vi "ATF_PID_V1.0.vi"() -> ()   [LabVIEW 2022 SP3]
panel:
  in  "Monitor":u16=1
  out "Boolean 783":bool
  out "C_FM_39":dbl format="%.2g"
  out "F_EPV_41":bool
  out "C_FM_9":dbl format="%.2g"
  in  "EXIT":bool
  out "F_PT_SC":dbl format="%.2g"
  out "Boolean 7":bool
  out "F_RTD_SC":dbl format="%.2g"
  out "F_PT_42":dbl format="%.2g"
  out "Boolean 781":bool
  out "Boolean 412":bool
  out "Boolean 201":bool
  out "F_PT_47":dbl format="%.2g"
  out "F_RTD_47":dbl format="%.2g"
  out "Boolean 959":bool
  out "Boolean 952":bool
  out "Boolean 780":bool
  out "Boolean 951":bool
  out "Boolean 950":bool
  out "Boolean 941":bool
  out "Boolean 945":bool
  out "Boolean 942":bool
  out "C_LS_LOX_Tank 23":u16(slide) scale=0.0..100.0
  out "G_PT_68":dbl format="%.2g"
  out "C_LS_LOX_Tank 24":u16(slide) scale=0.0..100.0
  out "M_PT_89":dbl format="%.2g"
  out "Boolean 779":bool
  out "Boolean 778":bool
  out "C_EPV_6":bool
  out "C_EPV_6 HSS":bool
  out "C_RTD_5":dbl format="%.2g"
  out "C_PT_5":dbl format="%.2g"
  out "Boolean 777":bool
  out "Boolean 776":bool
  out "C_EPV_13":bool
  out "C_EPV_13 HSS":bool
  out "Boolean 775":bool
  out "Boolean 845":bool
  out "Boolean 844":bool
  out "Boolean 774":bool
  out "Boolean 773":bool
  out "Boolean 873":bool
  out "Boolean 772":bool
  out "Boolean 771":bool
  out "Boolean 770":bool
  out "Boolean 769":bool
  out "Boolean 767":bool
  out "Boolean 766":bool
  out "F_EPV_45":bool
  out "F_EPV_45 HSS":bool
  out "Boolean 765":bool
  out "Boolean 727":bool
  out "Boolean 724":bool
  out "G_PT_72":dbl format="%.2g"
  out "M_PT_93":dbl format="%.2g"
  out "Boolean 1002":bool
  out "Boolean 998":bool
  out "Boolean 872":bool
  out "Boolean 871":bool
  out "Boolean 870":bool
  out "Boolean 862":bool
  out "Boolean 861":bool
  out "Boolean 860":bool
  out "Boolean 859":bool
  out "Boolean 830":bool
  out "I_PT_1":dbl format="%.2g"
  out "I_PT_2":dbl format="%.2g"
  out "E_PT_P2":dbl format="%.2g"
  out "E_PT_P1":dbl format="%.2g"
  out "Boolean 764":bool
  out "Boolean 763":bool
  out "N_EPV_8":bool
  out "Boolean 762":bool
  out "Boolean 761":bool
  out "Boolean 856":bool
  out "Boolean 843":bool
  out "C_PT_189":dbl format="%.2g"
  out "Boolean 791":bool
  out "Boolean 385":bool
  out "Boolean 212":bool
  out "Boolean 760":bool
  out "Boolean 759":bool
  out "Boolean 758":bool
  out "Boolean 757":bool
  out "Boolean 754":bool
  out "Boolean 1076":bool
  out "Boolean 1075":bool
  out "Boolean 958":bool
  out "Boolean 1074":bool
  out "Boolean 1072":bool
  out "Boolean 1073":bool
  out "Boolean 726":bool
  out "Boolean 901":bool
  out "Boolean 1071":bool
  out "Boolean 1033":bool
  out "Boolean 1027":bool
  out "Boolean 411":bool
  out "Boolean 897":bool
  out "Boolean 1070":bool
  out "Boolean 1069":bool
  out "Boolean 1042":bool
  out "Boolean 410":bool
  out "Boolean 1068":bool
  out "Boolean 1067":bool
  out "Boolean 1066":bool
  out "Boolean 1041":bool
  out "Boolean 1016":bool
  out "Boolean 896":bool
  out "Boolean 409":bool
  out "Boolean 1039":bool
  out "Boolean 1015":bool
  out "Boolean 1011":bool
  out "Boolean 1009":bool
  out "Boolean 982":bool
  out "Boolean 1065":bool
  out "Boolean 400":bool
  out "Boolean 408":bool
  out "N_PT_131":dbl format="%.2g"
  out "N_PT_193":dbl format="%.2g"
  out "N_PT_142":dbl format="%.2g"
  out "Boolean 894":bool
  out "Boolean 1063":bool
  out "Boolean 394":bool
  out "Boolean 393":bool
  out "Boolean 1058":bool
  out "Boolean 1018":bool
  out "Boolean 983":bool
  out "Boolean 1064":bool
  out "Boolean 981":bool
  out "Boolean 980":bool
  out "Boolean 979":bool
  out "Boolean 978":bool
  out "Boolean 1062":bool
  out "Boolean 1061":bool
  out "Boolean 977":bool
  out "Boolean 976":bool
  out "Boolean 975":bool
  out "Boolean 1060":bool
  out "Boolean 1059":bool
  out "Boolean 383":bool
  out "Boolean 1057":bool
  out "Boolean 391":bool
  out "Boolean 974":bool
  out "Boolean 883":bool
  out "Boolean 841":bool
  out "Boolean 864":bool
  out "Boolean 854":bool
  out "Boolean 846":bool
  out "Boolean 788":bool
  out "Boolean 796":bool
  out "Boolean 795":bool
  out "Boolean 789":bool
  out "Boolean 1056":bool
  out "Boolean 1055":bool
  out "Boolean 1054":bool
  out "Boolean 1053":bool
  out "Boolean 1052":bool
  out "Boolean 1051":bool
  out "Boolean 1050":bool
  out "Boolean 1049":bool
  out "Boolean 1048":bool
  out "Boolean 1047":bool
  out "Boolean 1046":bool
  out "Boolean 1045":bool
  out "Boolean 1044":bool
  out "Boolean 407":bool
  out "Boolean 1043":bool
  out "Boolean 957":bool
  out "Boolean 956":bool
  out "Boolean 955":bool
  out "Boolean 954":bool
  out "Boolean 953":bool
  out "Boolean 893":bool
  out "Boolean 969":bool
  out "Boolean 968":bool
  out "Boolean 967":bool
  out "Boolean 406":bool
  out "Boolean 966":bool
  out "Boolean 964":bool
  out "N_PT_118":dbl format="%.2g"
  out "Boolean 869":bool
  out "Boolean 1038":bool
  out "Boolean 972":bool
  out "Boolean 971":bool
  out "Boolean 970":bool
  out "Boolean 965":bool
  out "Boolean 868":bool
  out "Boolean 1037":bool
  out "Boolean 1036":bool
  out "Boolean 1035":bool
  out "Boolean 1034":bool
  out "N_PT_102":dbl format="%.2g"
  out "N_PT_107":dbl format="%.2g"
  out "Boolean 1032":bool
  out "Boolean 986":bool
  out "Boolean 1026":bool
  out "Boolean 1025":bool
  out "N_PT_149":dbl format="%.2g"
  out "Boolean 899":bool
  out "Boolean 985":bool
  out "Boolean 1024":bool
  out "Boolean 1023":bool
  out "Boolean 919":bool
  out "Boolean 918":bool
  out "Boolean 855":bool
  out "Boolean 800":bool
  out "Boolean 1022":bool
  out "Boolean 1021":bool
  out "Boolean 1020":bool
  out "Boolean 1019":bool
  out "Boolean 934":bool
  out "Boolean 835":bool
  out "Boolean 815":bool
  out "N_PT_201":dbl format="%.2g"
  out "Boolean 1007":bool
  out "Boolean 993":bool
  out "Boolean 984":bool
  out "Boolean 992":bool
  out "Boolean 991":bool
  out "M_PT_83":dbl format="%.2g"
  out "G_PT_63":dbl format="%.2g"
  out "N_PT_178":dbl format="%.2g"
  out "Boolean 847":bool
  out "Boolean 836":bool
  out "Boolean 211":bool
  out "Boolean 739":bool
  out "Boolean 802":bool
  out "M_EPV_90 HSS":bool
  out "G_EPV_69":bool
  out "M_EPV_90":bool
  out "G_EPV_69 HSS":bool
  out "Boolean 1017":bool
  out "Boolean 1013":bool
  out "Boolean 1010":bool
  out "Boolean 888":bool
  out "Boolean 398":bool
  out "Boolean 405":bool
  out "Boolean 1012":bool
  out "Boolean 1005":bool
  out "Boolean 1004":bool
  out "Boolean 887":bool
  out "Boolean 395":bool
  out "Boolean 404":bool
  out "Boolean 733":bool
  out "Boolean 9":bool
  out "Boolean 1003":bool
  out "Boolean 886":bool
  out "Boolean 995":bool
  out "C_LS_LOX_Tank 21":u16(slide) scale=0.0..100.0
  out "C_LS_LOX_Tank 22":u16(slide) scale=0.0..100.0
  out "Boolean 731":bool
  out "N_EPV_185":bool
  out "N_EPV_185 HSS":bool
  out "Boolean 8":bool
  out "Boolean 793":bool
  out "N_EPV_138":bool
  out "Boolean 748":bool
  out "N_EPV_138 HSS":bool
  out "Boolean 380":bool
  out "Boolean 999":bool
  out "Boolean 884":bool
  out "Boolean 994":bool
  out "Boolean 990":bool
  out "Boolean 989":bool
  out "Boolean 988":bool
  out "Boolean 987":bool
  out "M_PT_184":dbl format="%.2g"
  out "Boolean 831":bool
  out "N_PT_137":dbl format="%.2g"
  out "Boolean 402":bool
  out "Boolean 973":bool
  out "C_LS_LOX_Tank 20":u16(slide) scale=0.0..100.0
  out "Boolean 823":bool
  out "N_PT_123":dbl format="%.2g"
  out "C_LS_LOX_Tank 19":u16(slide) scale=0.0..100.0
  out "Boolean 822":bool
  out "N_PT_199":dbl format="%.2g"
  out "Boolean 943":bool
  out "Boolean 863":bool
  out "Boolean 382":bool
  out "Boolean 944":bool
  out "C_LS_LOX_Tank 18":u16(slide) scale=0.0..100.0
  out "Boolean 946":bool
  out "Boolean 947":bool
  out "Boolean 948":bool
  out "Boolean 949":bool
  out "Boolean 881":bool
  out "N_PT_207":dbl format="%.2g"
  out "Boolean 372":bool
  out "Boolean 931":bool
  out "Boolean 930":bool
  out "C_LS_LOX_Tank 17":u16(slide) scale=0.0..100.0
  out "Boolean 929":bool
  out "Boolean 928":bool
  out "Boolean 927":bool
  out "Boolean 926":bool
  out "Boolean 848":bool
  out "Boolean 922":bool
  out "Boolean 803":bool
  out "N_PT_170":dbl format="%.2g"
  out "N_PT_164":dbl format="%.2g"
  out "Boolean 829":bool
  out "Boolean 940":bool
  out "F_RTD_46":dbl format="%.2g"
  out "F_PT_46":dbl format="%.2g"
  out "Boolean 939":bool
  out "Boolean 938":bool
  out "Boolean 906":bool
  out "Boolean 937":bool
  out "Boolean 905":bool
  out "F_EPV_175":bool
  out "F_EPV_175 HSS":bool
  out "Boolean 865":bool
  out "Boolean 379":bool
  out "F_EPV_43":bool
  out "Boolean 853":bool
  out "Boolean 852":bool
  out "F_EPV_43 HSS":bool
  out "Boolean 209":bool
  out "Boolean 13":bool
  out "Boolean 851":bool
  out "Boolean 790":bool
  out "Boolean 756":bool
  out "Boolean 850":bool
  out "F_PT_41":dbl format="%.2g"
  out "Boolean 936":bool
  out "F_EPV_41 HSS":bool
  out "Boolean 208":bool
  out "Boolean 745":bool
  out "Boolean 378":bool
  out "Boolean 755":bool
  out "Boolean 753":bool
  out "Boolean 747":bool
  out "Boolean 746":bool
  out "N_EPV_72":bool
  out "N_EPV_72 HSS":bool
  out "Boolean 849":bool
  out "Boolean 744":bool
  out "F_EPV_38":bool
  out "Boolean 842":bool
  out "F_EPV_38 HSS":bool
  out "Boolean 720":bool
  out "Boolean 743":bool
  out "Boolean 740":bool
  out "Boolean 732":bool
  out "Boolean 925":bool
  out "Boolean 913":bool
  out "Boolean 898":bool
  out "Boolean 891":bool
  out "N_EPV_150":bool
  out "Boolean 699":bool
  out "N_EPV_150 HSS":bool
  out "Boolean 719":bool
  out "N_PT_151":dbl format="%.2g"
  out "Boolean 374":bool
  out "Boolean 373":bool
  out "Boolean 840":bool
  out "Boolean 725":bool
  out "D_PT_160":dbl format="%.2g"
  out "Boolean 838":bool
  out "Boolean 837":bool
  out "Boolean 834":bool
  out "Boolean 833":bool
  out "Boolean 832":bool
  out "Boolean 718":bool
  out "Boolean 714":bool
  out "Boolean 397":bool
  out "Boolean 6":bool
  out "Boolean 885":bool
  out "Boolean 874":bool
  out "C_LS_LOX_Tank 10":u16(slide) scale=0.0..100.0
  out "N_EPV_157 HSS":bool
  out "Boolean 5":bool
  out "N_EPV_157":bool
  out "Boolean 824":bool
  out "Boolean 710":bool
  out "C_EPV_14":bool
  out "Boolean 750":bool
  out "C_RTD_13":dbl format="%.2g"
  out "C_PT_13":dbl format="%.2g"
  out "Boolean 904":bool
  out "Boolean 858":bool
  out "N_EPV_128":bool
  out "N_EPV_128 HSS":bool
  out "Boolean 392":bool
  out "Boolean 370":bool
  out "Boolean 877":bool
  out "Boolean 202":bool
  out "Boolean 782":bool
  out "Boolean 4":bool
  out "Boolean 878":bool
  out "N_EPV_190":bool
  out "N_EPV_190 HSS":bool
  out "Boolean 839":bool
  out "Boolean 828":bool
  out "Boolean 768":bool
  out "Boolean 730":bool
  out "Boolean 729":bool
  out "C_PT_15":dbl format="%.2g"
  out "C_RTD_15":dbl format="%.2g"
  out "Boolean 827":bool
  out "Boolean 826":bool
  out "C_EPV_14 HSS":bool
  out "Boolean 12":bool
  out "C_EPV_125":bool
  out "C_EPV_125 HSS":bool
  out "C_RTD_SC":dbl format="%.2g"
  out "C_PT_SC":dbl format="%.2g"
  out "C_PT_12":dbl format="%.2g"
  out "Boolean 825":bool
  out "Boolean 818":bool
  out "C_RTD_12":dbl format="%.2g"
  out "C_EPV_3":bool
  out "Boolean 821":bool
  out "Boolean 752":bool
  out "Boolean 751":bool
  out "Boolean 749":bool
  out "Boolean 738":bool
  out "C_EPV_11":bool
  out "C_EPV_8":bool
  out "N_EPV_113":bool
  out "N_EPV_109":bool
  out "C_EPV_78":bool
  out "C_EPV_75":bool
  out "Boolean 742":bool
  out "Boolean 741":bool
  out "C_EPV_11 HSS":bool
  out "Boolean 363":bool
  out "C_EPV_3 HSS":bool
  out "Boolean 816":bool
  out "Boolean 11":bool
  out "Boolean 3":bool
  out "Boolean 813":bool
  out "Boolean 812":bool
  out "Boolean 736":bool
  out "Boolean 819":bool
  out "Boolean 814":bool
  out "C_EPV_8 HSS":bool
  out "C_RTD_8":dbl format="%.2g"
  out "Boolean 734":bool
  out "Boolean 200":bool
  out "Boolean 723":bool
  out "Boolean 722":bool
  out "N_EPV_8 HSS":bool
  out "Boolean 721":bool
  out "D_PT_115":dbl format="%.2g"
  out "Boolean 811":bool
  out "Boolean 810":bool
  out "Boolean 809":bool
  out "Boolean 808":bool
  out "Boolean 807":bool
  out "Boolean 384":bool
  out "Boolean 717":bool
  out "Boolean 716":bool
  out "Boolean 713":bool
  out "Boolean 711":bool
  out "Boolean 684":bool
  out "N_EPV_113 HSS":bool
  out "Boolean 712":bool
  out "C_PT_110":dbl format="%.2g"
  out "N_EPV_109 HSS":bool
  out "Boolean 366":bool
  out "Boolean 805":bool
  out "C_EPV_78 HSS":bool
  out "Boolean 804":bool
  out "Boolean 708":bool
  out "C_EPV_75 HSS":bool
  out "Boolean 707":bool
  out "Boolean 2":bool
  out "Boolean":bool
  out "Boolean 867":bool
  out "C_LS_LOX_Tank 8":u16(slide) scale=0.0..100.0
  out "Boolean 866":bool
  out "Boolean 735":bool
  out "Boolean 361":bool
  out "Boolean 199":bool
  out "Boolean 360":bool
  out "Boolean 198":bool
  out "EPV_ 21":bool
  out "N_EPV_CF1 HSS 21":bool
  # "SeCrTS Heavy- PID GUI"
  # "VERSION NUMBER :1.0"
  # "RELEASE DATE 08/07/2024"
  # "ATF Barrel"
  # "Surge Tank"
  # "Surge Tank"
  # "Surge Tank"
  # "Surge Tank"
  # "Surge Tank"
  # "Surge Tank"
  # "GN2"
  # "GN2"
  # "GN2"
  # "GN2"
  # "M_1"
  # "O2"
  # "GN2"
  # "GN2"
  # "GN2"
  # "GN2"
  # "Surge Tank"
  # "Surge Tank"
  # "ATF 400 L RUNTANK\nP:4MPa\nT:303K\nV:400L"
  # "LOX 400 L RUNTANK\nP:4MPa\nT:84K\nV:400L"
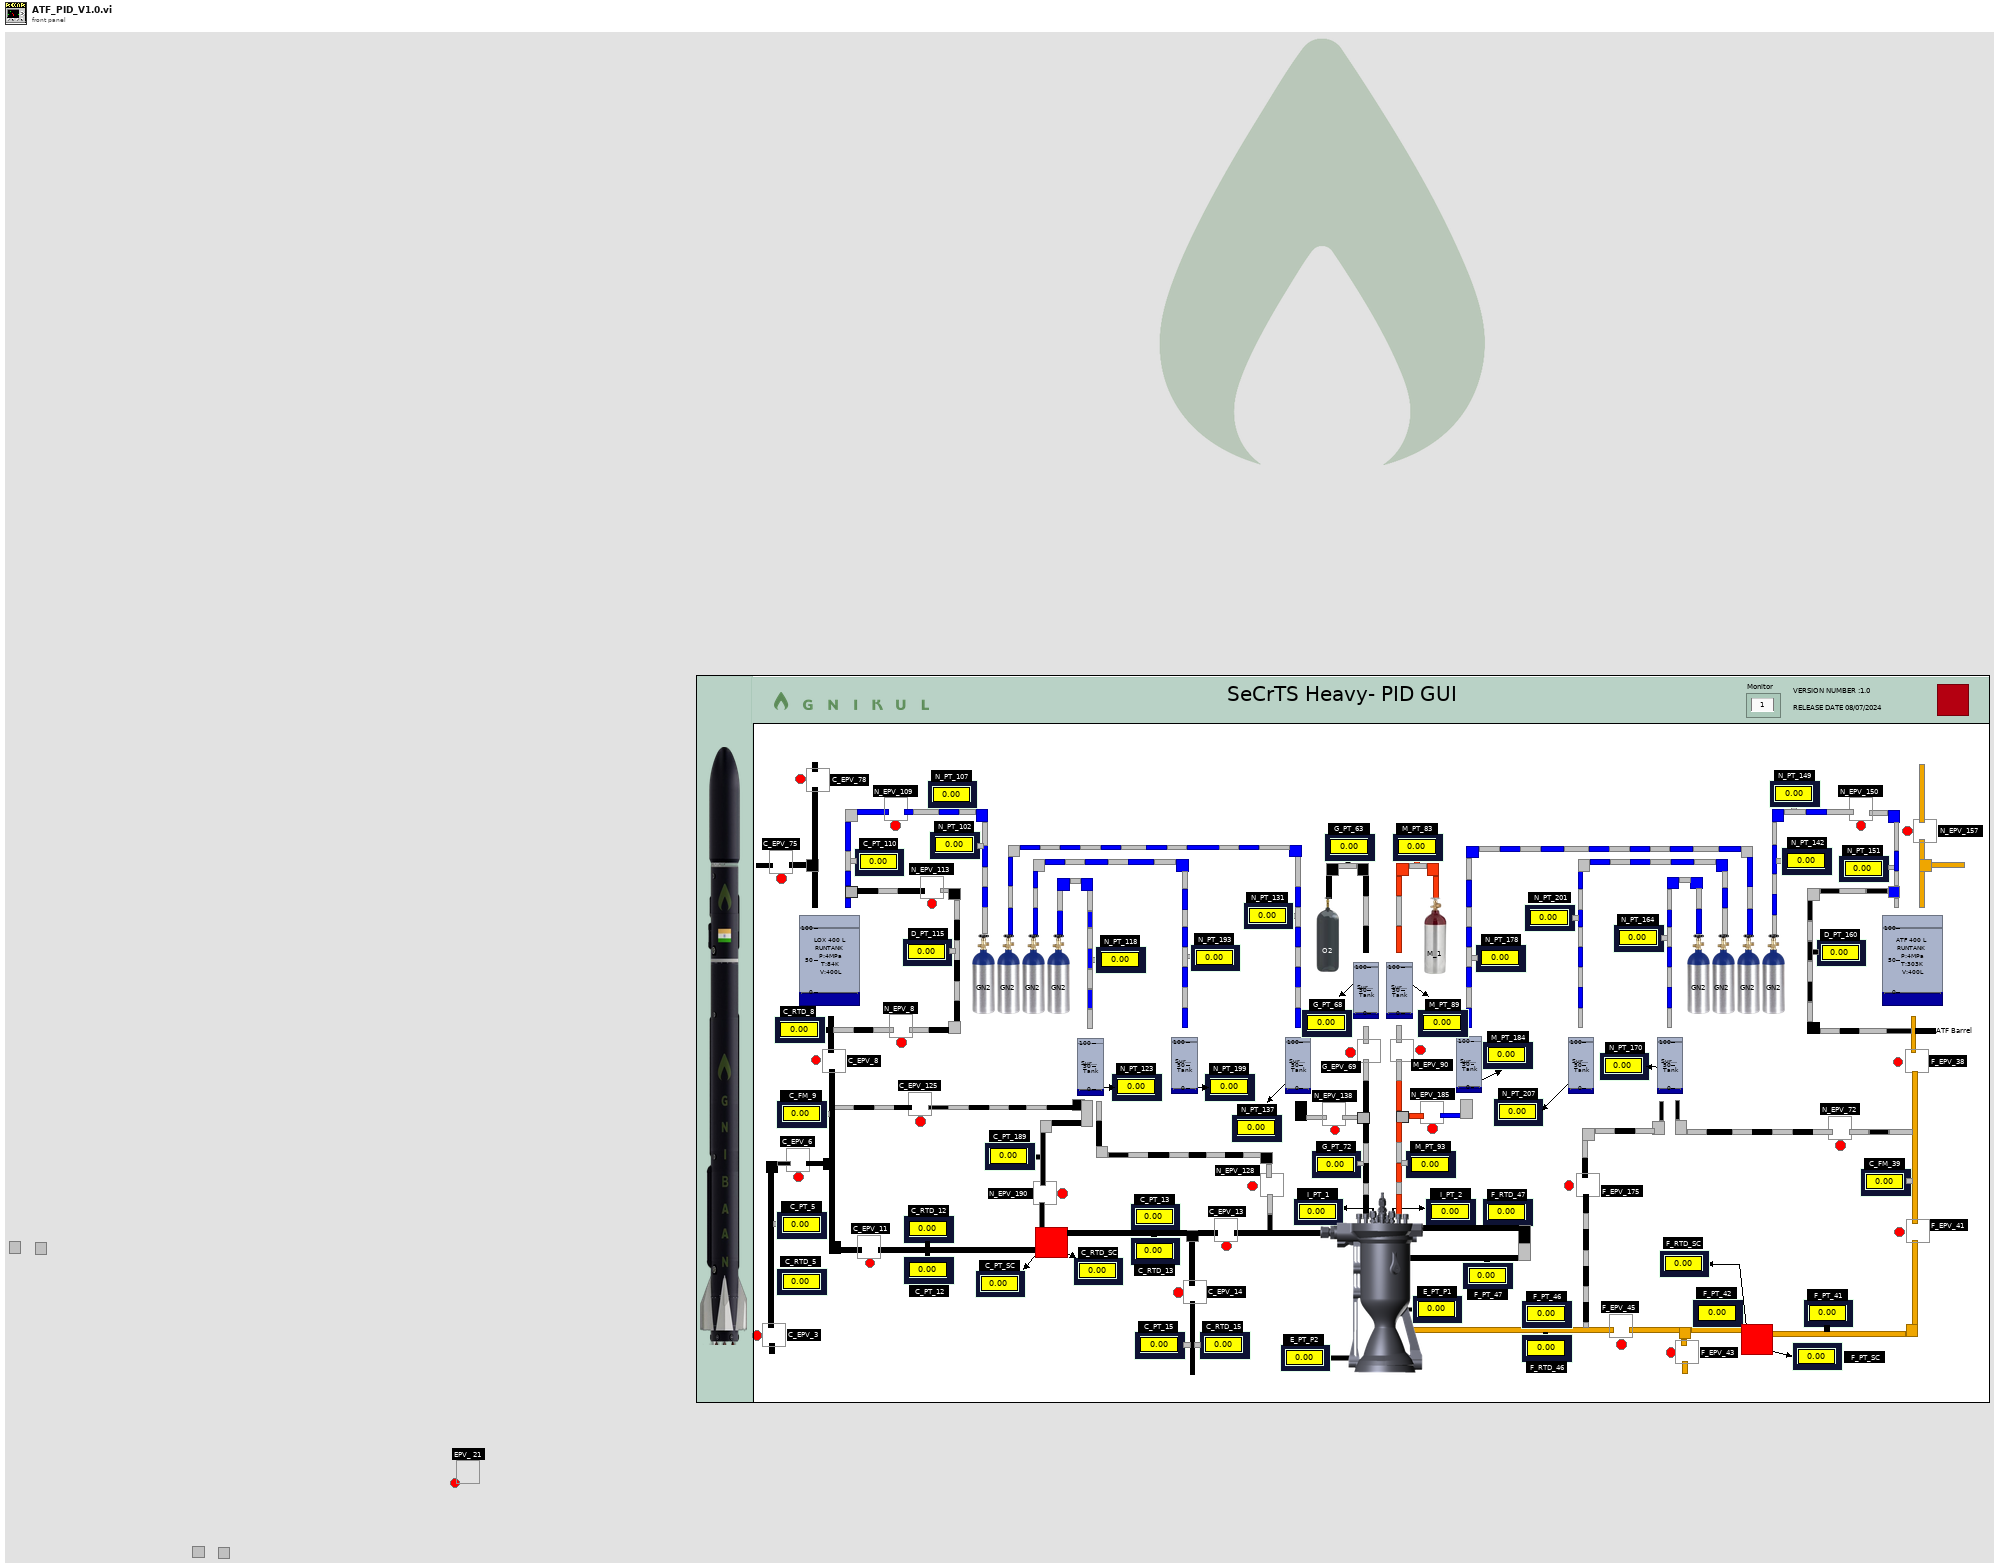
[diagram p1: front panel]
types:
  T1 = enum32{"Invalid", "Standard", "Closed", "Hidden", "Minimized", "Maximized"}
  T2 = typedef "SeCrTS-Notifier Ref.ctl" = cluster{"DO NOT S":refnum<notifier>, "AI V NOT P":refnum<notifier>, "AI C NOT S":refnum<notifier>, "TC NOT P":refnum<notifier>, "DI NOT S":refnum<notifier>, "DI NOT P":refnum<notifier>, "DO NOT P":refnum<notifier>, "AI C NOT  P":refnum<notifier>}
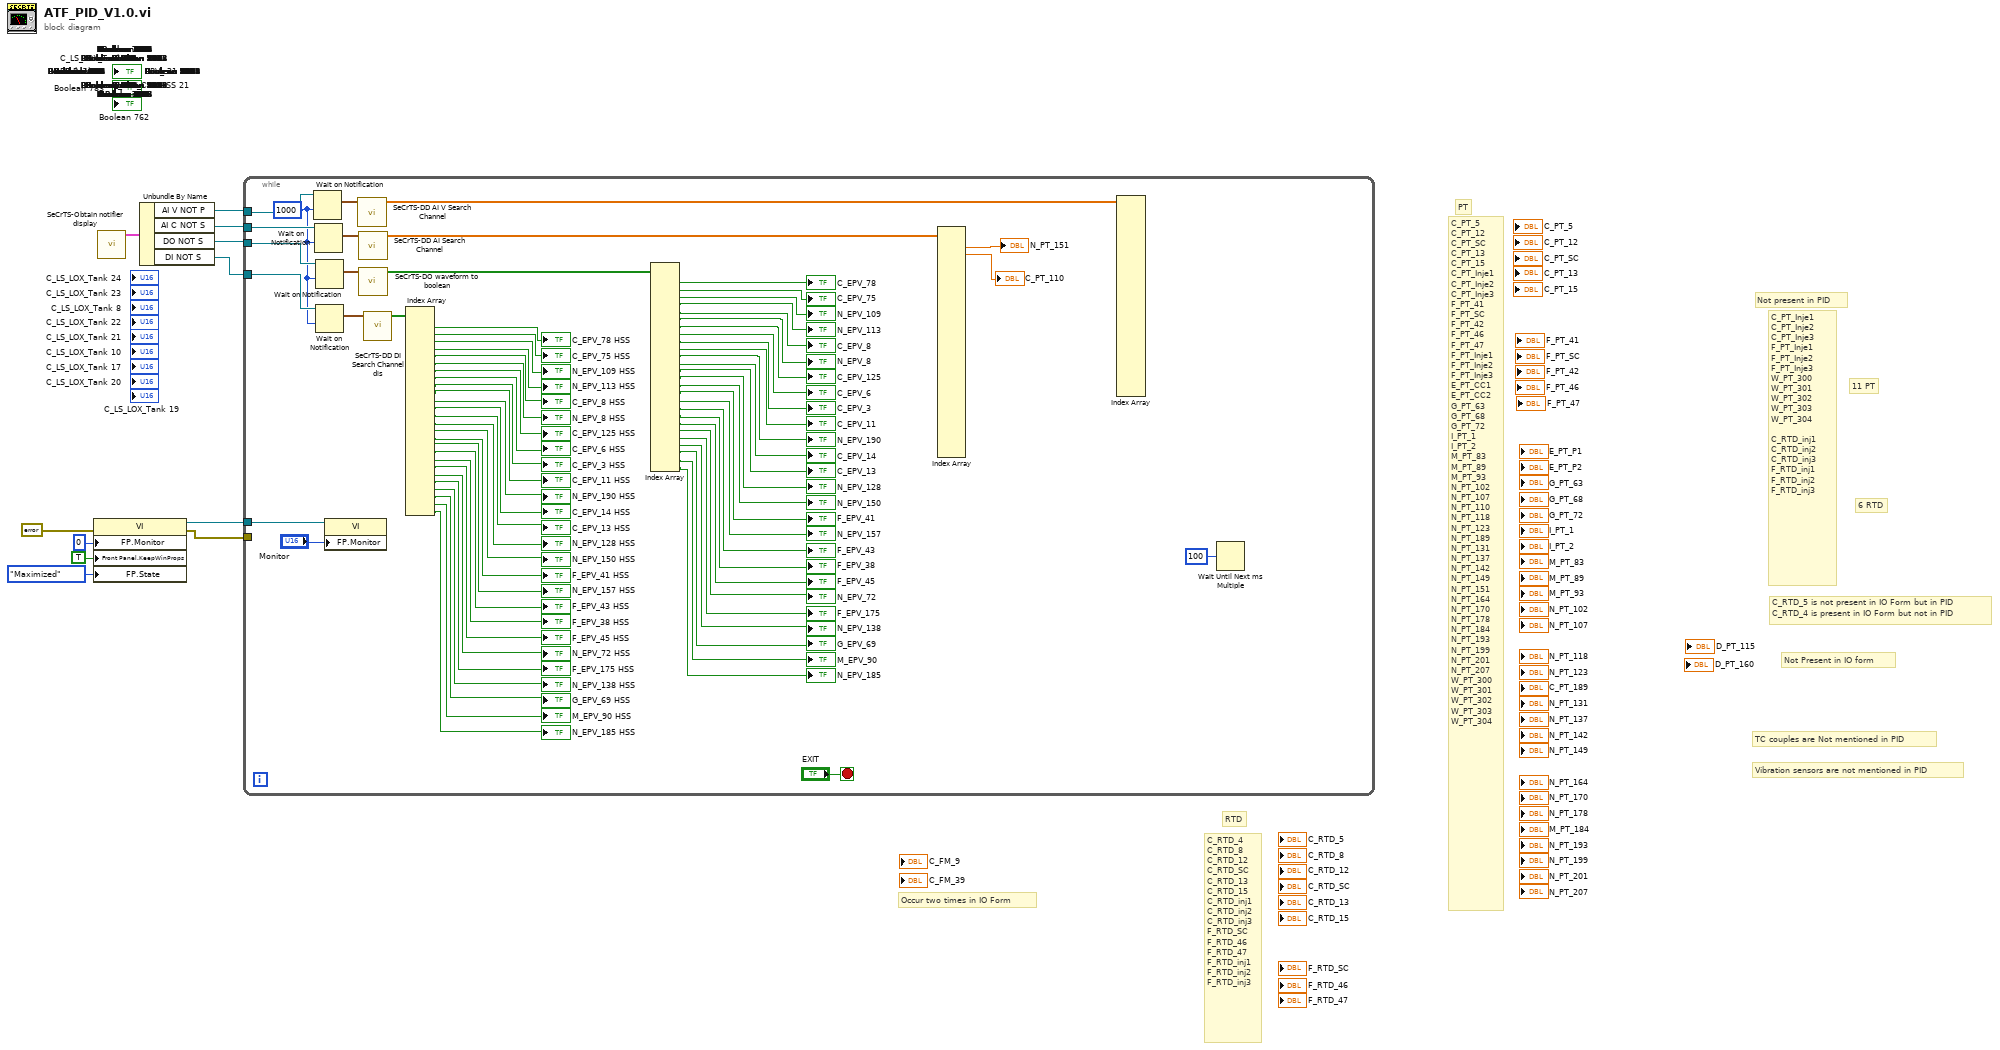
[diagram p0: block diagram]
diagram:
  # "Occur two times in IO Form"
  # "C_RTD_5 is not present in IO Form but in PID \nC_RTD_4 is present in IO Form but not in PID"
  # "Vibration sensors are not mentioned in PID"
  # "TC couples are Not mentioned in PID"
  # "11 PT"
  # "6 RTD"
  # "Not Present in IO form"
  # "Not present in PID"
  # "C_PT_Inje1\nC_PT_Inje2\nC_PT_Inje3\nF_PT_Inje1\nF_PT_Inje2\nF_PT_Inje3\nW_PT_300\nW_PT_301\nW_PT_302\nW_PT_303\nW_PT_304\n\nC_RTD_inj1\nC_RTD_inj2\nC_RTD_inj3\nF_RTD_inj1\nF_RTD_inj2\nF_RTD_inj3"
  # "RTD"
  # "C_RTD_4\nC_RTD_8\nC_RTD_12\nC_RTD_SC\nC_RTD_13\nC_RTD_15\nC_RTD_inj1\nC_RTD_inj2\nC_RTD_inj3\nF_RTD_SC\nF_RTD_46\nF_RTD_47\nF_RTD_inj1\nF_RTD_inj2\nF_RTD_inj3"
  # "PT"
  # "C_PT_5\nC_PT_12\nC_PT_SC\nC_PT_13\nC_PT_15\nC_PT_Inje1\nC_PT_Inje2\nC_PT_Inje3\nF_PT_41\nF_PT_SC\nF_PT_42\nF_PT_46\nF_PT_47\nF_PT_Inje1\nF_PT_Inje2\nF_PT_Inje3\nE_PT_CC1\nE_PT_CC2\nG_PT_63\nG_PT_68\nG_PT_72\nI_PT_1\nI_PT_2\nM_PT_83\nM_PT_89\nM_PT_93\nN_PT_102\nN_PT_107\nN_PT_110\nN_PT_118\nN_PT_123\nN_PT_189\nN_PT_131\nN_PT_137\nN_PT_142\nN_PT_149\nN_PT_151\nN_PT_164\nN_PT_170\nN_PT_178\nN_PT_184\nN_PT_193\nN_PT_199\nN_PT_201\nN_PT_207\nW_PT_300\nW_PT_301\nW_PT_302\nW_PT_303\nW_PT_304"
  n1 = property class="VI"(error in=errorcluster {"status"=FALSE, "code"=0, "source"=""} ("error in (no error)"), "FP.Monitor"=u16 0 ("Front Panel Window:Monitor"), "Front Panel.KeepWinProps"=TRUE ("Front Panel Window:Keep Window Proportions"), "FP.State"=T1."Maximized" ("Front Panel Window:State")) -> (reference out=w2:refnum<vi>, error out=w1:errorcluster)  [unwired: 1 in]
  n2 = call "SeCrTS-Obtain notifier display.vi"() -> ("NOT DIS Out"=w11:T2)  [unwired: 11 in]
  n3 = Unbundle By Name(w11) -> ("AI V NOT P"=w10:refnum<notifier>, "AI C NOT S"=w9:refnum<notifier>, "DO NOT S"=w8:refnum<notifier>, "DI NOT S"=w7:refnum<notifier>)
  n4 = while {
    tunnel: w10 -> [w77]
    tunnel: w9 -> [w80]
    tunnel: w8 -> [w74]
    tunnel: w7 -> [w73]
    tunnel: w2 -> [w15]
    tunnel: w1 -> [_]
    stop <- "EXIT" stop-if-true
    w16 = 1000 ("timeout in ms (-1)")
    n5 = Wait on Notification(notifier=w77, timeout in ms (-1)=w16) -> (notification=w76:waveform(dbl)[])  [unwired: 2 in, 3 out]
    n6 = Wait on Notification(notifier=w80, timeout in ms (-1)=w16) -> (notification=w79:waveform(dbl)[])  [unwired: 2 in, 3 out]
    n7 = Wait on Notification(notifier=w74, timeout in ms (-1)=w16) -> (notification=w70:waveform(dbl)[])  [unwired: 2 in, 3 out]
    n8 = Wait on Notification(notifier=w73, timeout in ms (-1)=w16) -> (notification=w72:digitalwaveform[])  [unwired: 2 in, 3 out]
    n9 = property class="VI"(reference=w15, "FP.Monitor"="Monitor") -> ()  [unwired: 1 in, 2 out]
    n10 = call "SeCrTS-DD AI V Search Channel.vi"("AI Data"=w76) -> ("FeedBack"=w75:dbl[])  [unwired: 10 in]
    n11 = call "SeCrTS-DD AI Search Channel.vi"("AI Data"=w79) -> ("FeedBack"=w78:dbl[])  [unwired: 10 in]
    n12 = call "SeCrTS-DO waveform to boolean.vi"("DO"=w70) -> ("DO"=w69:bool[])  [unwired: 10 in]
    n13 = call "SeCrTS-DD DI Search Channel dis.vi"("DI Data"=w72) -> ("Array 2"=w71:bool[])  [unwired: 10 in]
    n14 = Index Array(array=w71) -> (element #1=→"C_EPV_78 HSS":bool, element #2=→"C_EPV_75 HSS":bool, element #3=→"N_EPV_109 HSS":bool, element #4=→"N_EPV_113 HSS":bool, element #5=→"C_EPV_8 HSS":bool, element #6=→"N_EPV_8 HSS":bool, element #7=→"C_EPV_125 HSS":bool, element #8=→"C_EPV_6 HSS":bool, element #9=→"C_EPV_3 HSS":bool, element #10=→"C_EPV_11 HSS":bool, element #11=→"N_EPV_190 HSS":bool, element #12=→"C_EPV_14 HSS":bool, element #13=→"C_EPV_13 HSS":bool, element #14=→"N_EPV_128 HSS":bool, element #15=→"N_EPV_150 HSS":bool, element #16=→"F_EPV_41 HSS":bool, element #17=→"N_EPV_157 HSS":bool, element #18=→"F_EPV_43 HSS":bool, element #19=→"F_EPV_38 HSS":bool, element #20=→"F_EPV_45 HSS":bool, element #21=→"N_EPV_72 HSS":bool, element #22=→"F_EPV_175 HSS":bool, element #23=→"N_EPV_138 HSS":bool, element #24=→"G_EPV_69 HSS":bool, element #25=→"M_EPV_90 HSS":bool, element #26=→"N_EPV_185 HSS":bool)  [unwired: 26 in]
    n15 = Index Array(array=w69) -> (element #1=→"C_EPV_78":bool, element #2=→"C_EPV_75":bool, element #3=→"N_EPV_109":bool, element #4=→"N_EPV_113":bool, element #5=→"C_EPV_8":bool, element #6=→"N_EPV_8":bool, element #7=→"C_EPV_125":bool, element #8=→"C_EPV_6":bool, element #9=→"C_EPV_3":bool, element #10=→"C_EPV_11":bool, element #11=→"N_EPV_190":bool, element #12=→"C_EPV_14":bool, element #13=→"C_EPV_13":bool, element #14=→"N_EPV_128":bool, element #15=→"N_EPV_150":bool, element #16=→"F_EPV_41":bool, element #17=→"N_EPV_157":bool, element #18=→"F_EPV_43":bool, element #19=→"F_EPV_38":bool, element #20=→"F_EPV_45":bool, element #21=→"N_EPV_72":bool, element #22=→"F_EPV_175":bool, element #23=→"N_EPV_138":bool, element #24=→"G_EPV_69":bool, element #25=→"M_EPV_90":bool, element #26=→"N_EPV_185":bool)  [unwired: 26 in]
    n16 = Index Array(array=w78) -> (element #1=→"N_PT_151":dbl, element #2=→"C_PT_110":dbl)  [unwired: 29 in, 27 out]
    n17 = Index Array(array=w75) -> ()  [unwired: 25 in, 25 out]
    n18 = Wait Until Next ms Multiple(millisecond multiple=u32 100) -> ()  [unwired: 1 out]
  }
